vi "Check.vi"(8 "error in (no error)":errorcluster, 11 "Queue Name":string) -> (0 "error out":errorcluster)   [LabVIEW 2019, in "ADLINK Motion Card.lvlib"]
uses:
  ADLINK Motion Card.lvlib
  Queues/Message Cluster.ctl
  Queues/Queues.lvlib
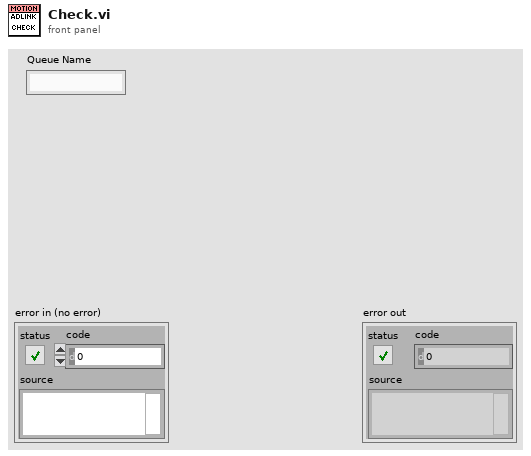
[diagram p1: front panel]
types:
  T1 = typedef "Queues.lvlib/Message Cluster.ctl" = cluster{"State":string, "Data":variant}
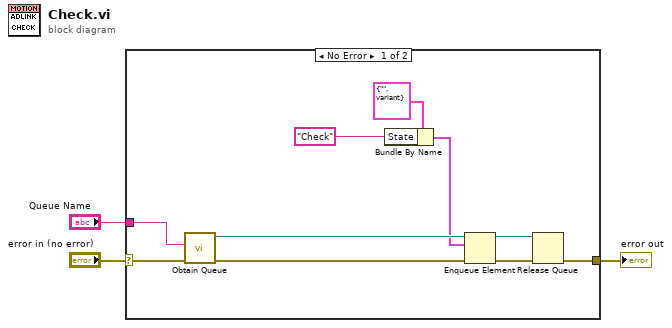
[diagram p0: block diagram]
diagram:
  n1 = case shown="No Error" "error in (no error)" {
    selector: "error in (no error)" -> [w12 w14]
    tunnel: "Queue Name" -> [w13 _]
    tunnel: [w5 w14] -> w1
    frame No Error {
      n2 = call "Obtain Queue.vi"("Error In"=w12, "Queue Name"=w13) -> ("Error Out"=w11:errorcluster, "queue out"=w10:refnum<queue>)  [unwired: 8 in]
      n3 = Bundle By Name(cluster=T1 {"State"="", "Data"=variant} ("element"), "State"="Check") -> (w8:T1)
      n4 = Enqueue Element(queue=w10, element=w8, error in (no error)=w11) -> (queue out=w6:refnum<queue>, error out=w7:errorcluster)  [unwired: 1 in, 1 out]
      n5 = Release Queue(queue=w6, error in (no error)=w7) -> (error out=w5:errorcluster)  [unwired: 1 in, 2 out]
    }
    frame Error {
    }
  }
  "error out" <- w1
